vi "Maps-Initialization.vi"(0 "Automation Refnum in":refnum<k7>, 7 "URL":string="https://maps.googleapis.com/maps/api/staticmap", 11 "error in (no error)":errorcluster) -> (4 "Google Maps Resource Out":T1, 15 "error out":errorcluster)   [LabVIEW 2020]
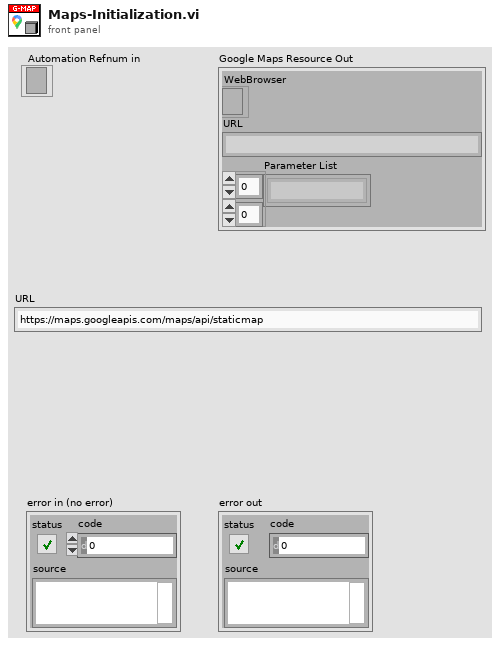
[diagram p1: front panel]
types:
  T1 = cluster{"WebBrowser":refnum<k7>, "URL":string, "Parameter List":string[][]}
  T2 = cluster{"Automation Refnum in":refnum<k7>, "URL":string, "Parameter List":string[][]}
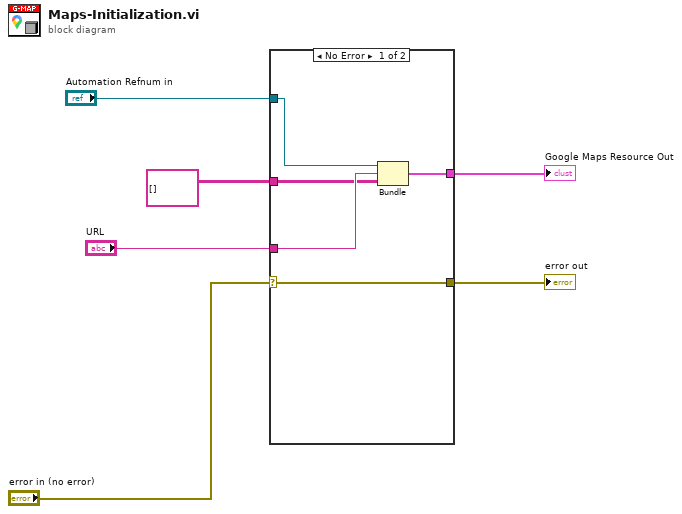
[diagram p0: block diagram]
diagram:
  n1 = case shown="No Error" "error in (no error)" {
    selector: "error in (no error)" -> [w7 w12]
    tunnel: "Automation Refnum in" -> [w11 _]
    tunnel: "URL" -> [w10 _]
    tunnel: [w9 _] -> w3
    tunnel: string[][] [] ("Parameter List") -> [w8 _]
    tunnel: [w7 w12] -> w6
    frame No Error {
      n2 = Bundle("Automation Refnum in"=w11, "URL"=w10, "Parameter List"=w8) -> (w9:T2)  [unwired: 1 in]
    }
    frame Error {
    }
  }
  "error out" <- w6
  "Google Maps Resource Out" <- w3
